vi "Script Init Msg Input.vi"(8 "error in":errorcluster, 9 "Name Msg Refs.Init Msg VI":refnum<vi>, 10 "Terminal Attributes (Init Msg Input)":T1) -> (0 "error out":errorcluster)   [LabVIEW 2025, in "_Rescript.lvlib" / "Msg.lvlib" / "Msg.lvclass"]
uses:
  Msg.lvclass
  Terminal Attributes.ctl
  Attributes.ctl
  <vilib>/Utility/traverseref.llb/TRef TravTarget.ctl
  Msg.lvclass/Msg.ctl
  _Rescript.lvlib
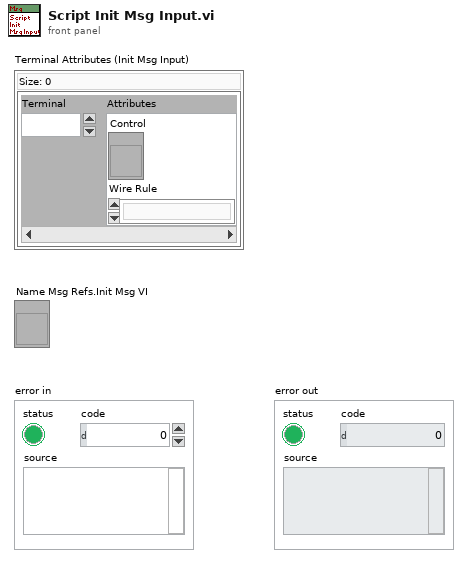
[diagram p1: front panel]
types:
  T1 = typedef "_Rescript.lvlib/Terminal Attributes.ctl" = map{i32, T2}
  T2 = typedef "_Rescript.lvlib/Attributes.ctl" = cluster{"Control":refnum<vi>, "Wire Rule":enum16{"Invalid Wire Rule", "Required", "Recommended", "Optional", "Dynamic Dispatch"}}
  T3 = typedef "TRef TravTarget.ctl" = enum16{"FP", "BD", "Other"}
  T4 = enum16{"Invalid Wire Rule", "Required", "Recommended", "Optional", "Dynamic Dispatch"}
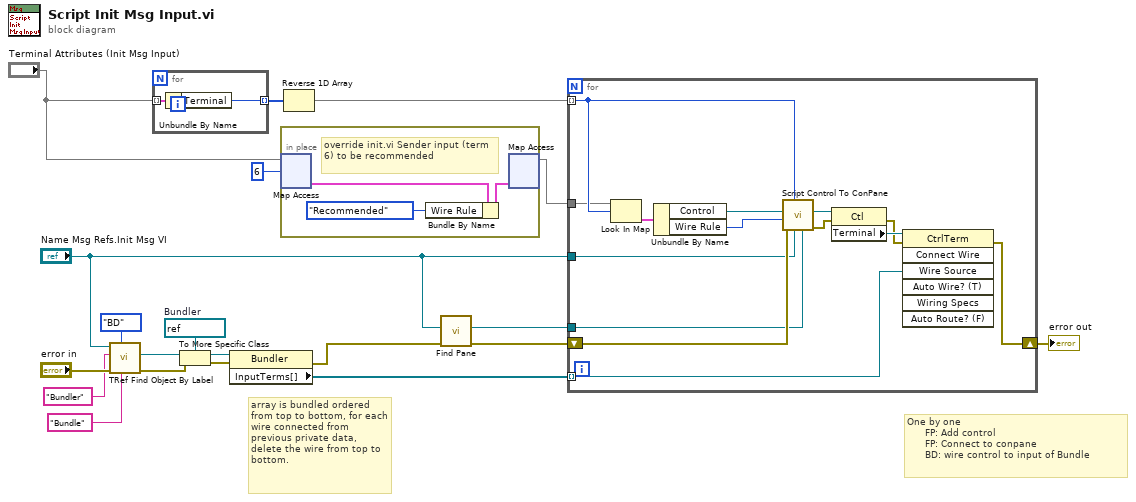
[diagram p0: block diagram]
diagram:
  w14 = refnum<vi> refnum  # Bundler
  # "array is bundled ordered from top to bottom, for each wire connected from previous private data, delete the wire from top to bottom."
  # "One by one\n      FP: Add control\n      FP: Connect to conpane\n      BD: wire control to input of Bundle"
  n1 = call <vilib>:"TRef Find Object By Label.vi"("Label"="Bundle", "Traverse Target"=TRef_TravTarget."BD", "error in (no error)"="error in", "Class Name"="Bundler", "VI Ref"="Name Msg Refs.Init Msg VI") -> ("error out"=w18:errorcluster, "Found Obj Ref"=w17:refnum<vi>)  [unwired: 3 in, 2 out]
  n2 = for {
    tunnel: "Terminal Attributes (Init Msg Input)" -> [w22] mode=indexing
    tunnel: [w21] -> w20 mode=indexing
    n3 = Unbundle By Name(w22) -> ("Terminal"=w21:i32)
  }
  n4 = To More Specific Class(target class=w14, reference=w17, error in=w18) -> (specific class reference=w12:refnum<vi>, error out=w11:errorcluster)
  n5 = property class="Bundler"(reference=w12, error in=w11) -> (error out=w3:errorcluster, "InputTerms[]"=w8:refnum<vi>[])  [unwired: 1 out]
  n6 = in-place {
    # "override init.vi Sender input (term 6) to be recommended"
    n7 = in-place-map #1("Terminal Attributes (Init Msg Input)", 6 ("Terminal Index")) -> (w25:T2)  [unwired: 1 in, 1 out]
    n8 = Bundle By Name(cluster=w25, "Wire Rule"=T4."Recommended") -> (w24:T2)
    n9 = in-place-map #1(w24) -> (w7:T1)  [unwired: 1 in, 2 out]
  }
  n10 = Reverse 1D Array(array=w20) -> (reversed array=w19:i32[])
  n11 = call "Find Pane.vi"("error in"=w3, "VI Ref"="Name Msg Refs.Init Msg VI") -> ("error out"=w2:errorcluster, "Pane Ref"=w5:refnum<vi>)  [unwired: 8 in]
  n12 = for {
    tunnel: w19 -> [w27] mode=indexing
    tunnel: w7 -> [w26]
    tunnel: w5 -> [w32]
    tunnel: "Name Msg Refs.Init Msg VI" -> [w31]
    tunnel: w8 -> [w38] mode=indexing
    shift-right: [w36] -> w9
    shift-left: w2 -> [w33]
    n13 = Look In Map(map=w26, key=w27) -> (value=w30:T2)  [unwired: 1 in, 1 out]
    n14 = Unbundle By Name(w30) -> ("Control"=w29:refnum<vi>, "Wire Rule"=w28:T4)
    n15 = call "Script Control To ConPane.vi"("Pane"=w32, "VI Ref"=w31, "Terminal"=w27, "error in"=w33, "Wire Rule"=w28, "Control To Duplicate"=w29) -> ("error out"=w34:errorcluster, "Duplicated Control"=w35:refnum<vi>)  [unwired: 4 in]
    n16 = property class="Ctl"(reference=w35, error in=w34) -> (error out=w37:errorcluster, "Terminal"=w39:refnum<vi>)  [unwired: 1 out]
    n17 = invoke class="CtrlTerm" method="Connect Wire"(reference=w39, error in=w37, "Wire Source"=w38) -> (error out=w36:errorcluster)  [unwired: 4 in, 6 out]
  }
  "error out" <- w9
